vi "Send Trigger.vi"(8 "error in (no error)":errorcluster, 9 "Wait for OPC (F: Do not Wait)":bool, 10 "Ignore Trigger Source (F: Do not Ignore)":bool, 11 "VISA resource name":refnum<visa-resource-name>) -> (0 "error out":errorcluster, 3 "VISA resource name out":refnum<visa-resource-name>)   [LabVIEW 2023, in "Agilent ENA Series.lvlib"]
doc: "Configures trigger."
uses:
  Agilent ENA Series.lvlib
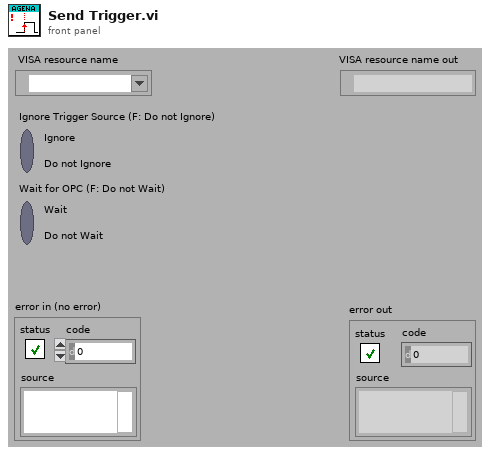
[diagram p1: front panel]
types:
  T1 = cluster{"Status":bool, "Code":i32, "Source (VI Name)":string}
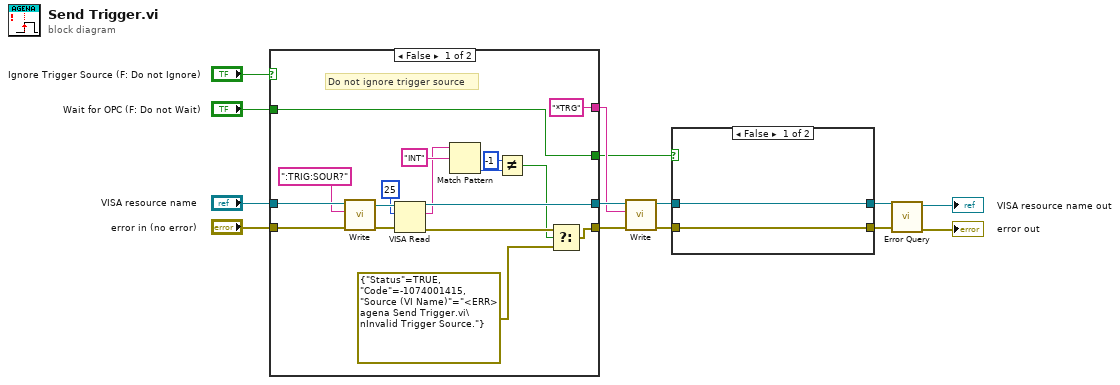
[diagram p0: block diagram]
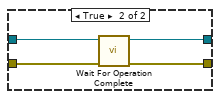
[diagram p2: hidden frame]
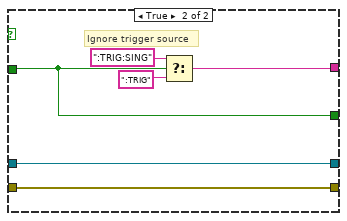
[diagram p3: hidden frame]
diagram:
  n1 = case shown="False" "Ignore Trigger Source (F: Do not Ignore)" {
    tunnel: "Wait for OPC (F: Do not Wait)" -> [w15 w32]
    tunnel: ["*TRG" w35] -> w9
    tunnel: "VISA resource name" -> [w30 w34]
    tunnel: "error in (no error)" -> [w29 w33]
    tunnel: [w24 w34] -> w10
    tunnel: [w23 w33] -> w11
    tunnel: [w15 w32] -> w1
    frame False {
      # "Do not ignore trigger source"
      n2 = call "Write.vi"("error in (no error)"=w29, "String ()"=":TRIG:SOUR?", "VISA resource name"=w30) -> ("error out"=w28:errorcluster, "VISA resource name out"=w27:refnum<visa-resource-name>)  [unwired: 6 in, 1 out]
      n3 = VISA Read(VISA resource name=w27, byte count=u32 25, error in (no error)=w28) -> (VISA resource name out=w24:refnum<visa-resource-name>, read buffer=w17:string, error out=w21:errorcluster)  [unwired: 1 out]
      n4 = Match Pattern(string=w17, regular expression="INT" ("x")) -> (offset past match=w19:i32)  [unwired: 1 in, 3 out]
      n5 = Not Equal?(x=-1, y=w19) -> (x != y?=w16:bool)
      n6 = Select(t=w21, s=w16, f=T1 {"Status"=TRUE, "Code"=-1074001415, "Source (VI Name)"="<ERR> agena Send Trigger.vi\nInvalid Trigger Source."}) -> (s? t:f=w23:T1)
    }
    frame True {
      # "Ignore trigger source"
      n7 = Select(t=":TRIG:SING", s=w32, f=":TRIG") -> (s? t:f=w35:string)
    }
  }
  n8 = call "Write.vi"("error in (no error)"=w11, "String ()"=w9, "VISA resource name"=w10) -> ("error out"=w4:errorcluster, "VISA resource name out"=w5:refnum<visa-resource-name>)  [unwired: 6 in, 1 out]
  n9 = case shown="False" w1 {
    tunnel: w5 -> [w39 w43]
    tunnel: w4 -> [w38 w42]
    tunnel: [w39 w41] -> w3
    tunnel: [w38 w40] -> w2
    frame False {
    }
    frame True {
      n10 = call "Wait For Operation Complete.vi"("error in (no error)"=w42, "VISA resource name"=w43) -> ("error out"=w40:errorcluster, "VISA resource name out"=w41:refnum<visa-resource-name>)  [unwired: 8 in]
    }
  }
  n11 = call "Error Query.vi"("error in (no error)"=w2, "VISA resource name"=w3) -> ("error out"=→"error out":errorcluster, "VISA resource name out"=→"VISA resource name out":refnum<visa-resource-name>)  [unwired: 6 in, 2 out]
